vi "CompareFloatArray.vi"(10 "destination":dbl[](array[numeric]), 11 "source":dbl[](array[numeric])) -> (3 "equal":bool)   [LabVIEW 2018]
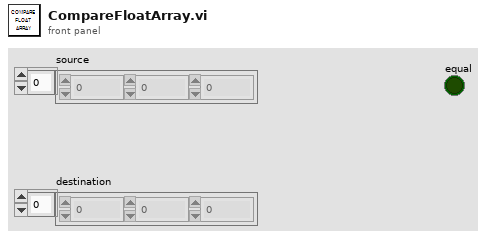
[diagram p1: front panel]
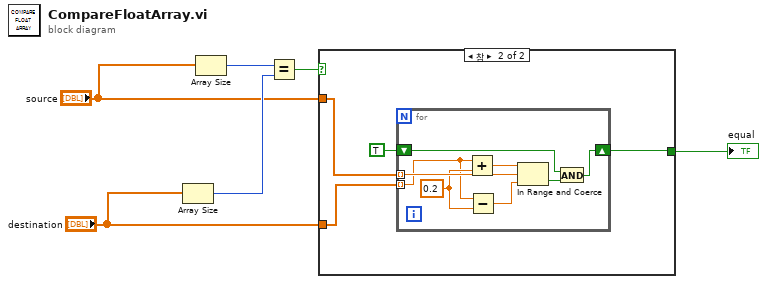
[diagram p0: block diagram]
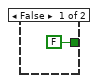
[diagram p2: hidden frame]
diagram:
  n1 = Array Size(array="destination") -> (size(s)=w5:i32)
  n2 = Array Size(array="source") -> (size(s)=w6:i32)
  n3 = Equal?(x=w6, y=w5) -> (x = y?=w4:bool)
  n4 = case shown="참" w4 {
    tunnel: "source" -> [_ w10]
    tunnel: "destination" -> [_ w9]
    tunnel: [FALSE w8] -> w1
    frame False {
    }
    frame True {
      n5 = for {
        tunnel: w10 -> [w17] mode=indexing
        shift-right: [w18] -> w8
        shift-left: TRUE -> [w19]
        tunnel: w9 -> [w15] mode=indexing
        w16 = 0.2
        n6 = Add(x=w15, y=w16) -> (x+y=w14:dbl)
        n7 = Subtract(x=w15, y=w16) -> (x-y=w13:dbl)
        n8 = In Range and Coerce(upper limit=w14, x=w17, lower limit=w13) -> (In Range?=w12:bool)  [unwired: 1 out]
        n9 = And(x=w19, y=w12) -> (x .and. y?=w18:bool)
      }
    }
  }
  "equal" <- w1
